vi "Close Param.vi"(8 "error in (no error)":errorcluster, 11 "Param in":T1) -> (0 "error out":errorcluster)   [LabVIEW 2019, in "Inputs.lvlib"]
uses:
  Inputs.lvlib
  Ctl/Param.ctl
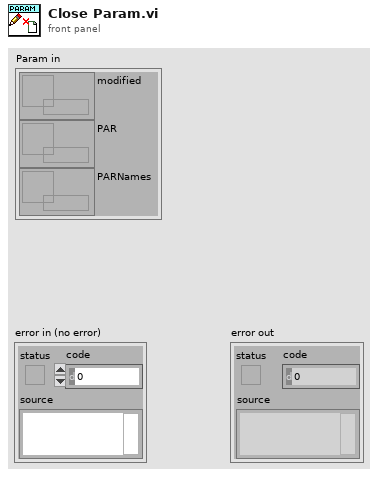
[diagram p1: front panel]
types:
  T1 = typedef "Inputs.lvlib/Param.ctl" = cluster{"modified":refnum<data-value>, "PAR":refnum<data-value>, "PARNames":refnum<data-value>}
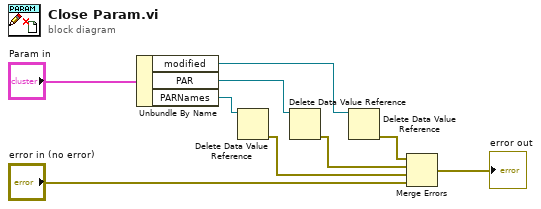
[diagram p0: block diagram]
diagram:
  n1 = Unbundle By Name("Param in") -> ("modified"=w9:refnum<data-value>, "PAR"=w7:refnum<data-value>, "PARNames"=w6:refnum<data-value>)
  n2 = Delete Data Value Reference(data value reference=w6) -> (error out=w4:errorcluster)  [unwired: 1 in, 1 out]
  n3 = Delete Data Value Reference(data value reference=w7) -> (error out=w5:errorcluster)  [unwired: 1 in, 1 out]
  n4 = Delete Data Value Reference(data value reference=w9) -> (error out=w8:errorcluster)  [unwired: 1 in, 1 out]
  n5 = Merge Errors(w8, w5, w4, "error in (no error)") -> (→"error out":errorcluster)
